vi "Config Trigger.vi"(2 "Scope Model":T1=enum."Tek TDS 694C", 4 "Trigger Coupling":i32(ring)=1 items=["main trigger", "DC", "noise reject"], 5 "Trigger Slope":i32(ring) items=["Positive", "Negative"], 6 "Trigger Level (V)":dbl, 7 "error in (no error)":errorcluster, 8 "Trigger Source":u16(ring) items=["Ch. 01", "Ch 02", "Ch. 03", "Ch. 04", "Aux"], 9 "Trigger Type":u16(ring)=1 items=["Auto", "Normal"], 10 "Scope Address":refnum<visa-resource-name>) -> (0 "error out":errorcluster, 3 "reference out":refnum<visa-resource-name>)   [LabVIEW 2020]
uses:
  Typedefs/Scope Models.ctl
  <instrlib>/tktds7xx/tktds7xx.llb/TKTDS 7XX Trigger Mode/Holdoff.vi
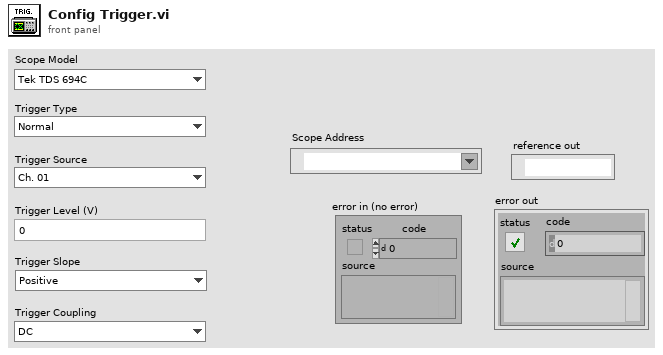
[diagram p1: front panel]
types:
  T1 = typedef "Scope Models.ctl" = enum16{"Tek TDS 684A/B/C", "Tek TDS 694C", "Tek TDS 744/A", "Tek TDS 754A/C/D", "Tek TDS 784A/C/D"}
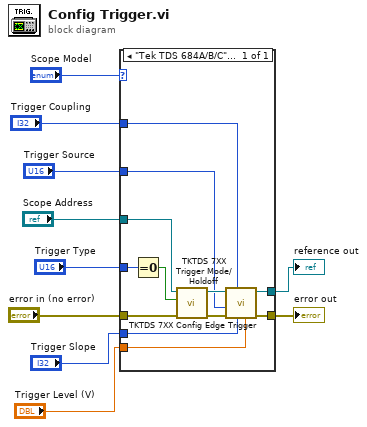
[diagram p0: block diagram]
diagram:
  n1 = case shown="\"Tek TDS 684A/B/C\", Default" "Scope Model" {
    tunnel: "Trigger Type" -> [w22]
    tunnel: "Trigger Source" -> [w18]
    tunnel: "Trigger Coupling" -> [w17]
    tunnel: "Trigger Level (V)" -> [w16]
    tunnel: "Trigger Slope" -> [w15]
    tunnel: "Scope Address" -> [w14]
    tunnel: "error in (no error)" -> [w13]
    tunnel: [w12] -> w3
    tunnel: [w11] -> w2
    frame "Tek TDS 684A/B/C", Default {
      n2 = Equal To 0?(x=w22) -> (x = 0?=w21:bool)
      n3 = call "TKTDS 7XX Trigger Mode/Holdoff.vi"("error in (no error)"=w13, "trigger mode (T:auto)"=w21, "VISA session"=w14) -> ("error out"=w19:errorcluster, "dup VISA session"=w20:refnum<visa-resource-name>)  [unwired: 6 in, 1 out]
      n4 = call <instrlib>:"TKTDS 7XX Config Edge Trigger.vi"("voltage level"=w16, "trigger slope (pos:0)"=w15, "trigger coupling (DC:1)"=w17, "error in (no error)"=w19, "trigger source (ch1:0)"=w18, "VISA session"=w20) -> ("error out"=w11:errorcluster, "dup VISA session"=w12:refnum<visa-resource-name>)  [unwired: 4 in]
    }
  }
  "error out" <- w2
  "reference out" <- w3
